vi "F8588A Read Stream.vi"(7 "read timeout [ms] (30000s)":u32=30000, 8 "error in (no error)":errorcluster, 9 "sample size [B]":i32=2, 10 "samples count":i32, 11 "VISA session":refnum<visa-resource-name>) -> (0 "error out":errorcluster, 1 "waveform data int32":i32[](array[numeric]), 2 "waveform data [V]":dbl[](array[numeric]), 3 "dup VISA session":refnum<visa-resource-name>, 4 "scale factor":dbl, 6 "read samples":i32)   [LabVIEW 2020]
doc: "Reads digitized data from memory. If 'Max Read' is set to -1 it reads all available data. It should work with SINt, DINT, SREAL and DREAL modes. ASCII read mode is not finished. It selects the OFORMAT automaticlaly. Data are returned already scaled if transfered in INT."
uses:
  d273381f-8530-47b4-8073-8e484cff5eca.vi
  <vilib>/Utility/error.llb/Error Cluster From Error Code.vi
  <vilib>/ErrorRing/Error Ring.xnode
panel:
  out "reading loop iteration":i32
  out "expected data length (w/o LF)":u32
  out "data length":i32
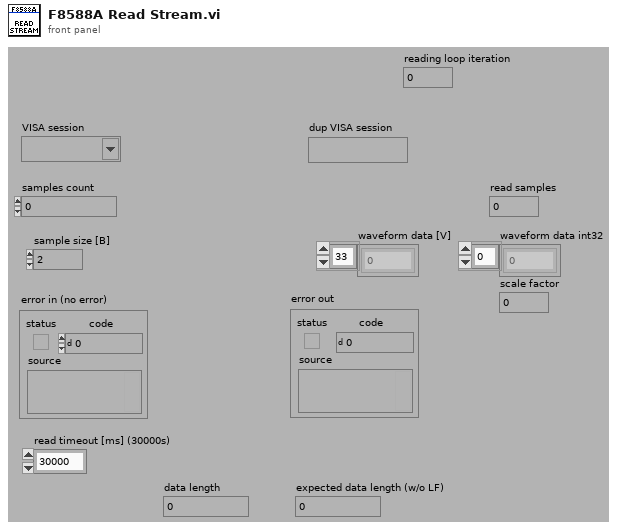
[diagram p1: front panel]
types:
  T1 = enum16{"big-endian, network order", "native, host order", "little-endian"}
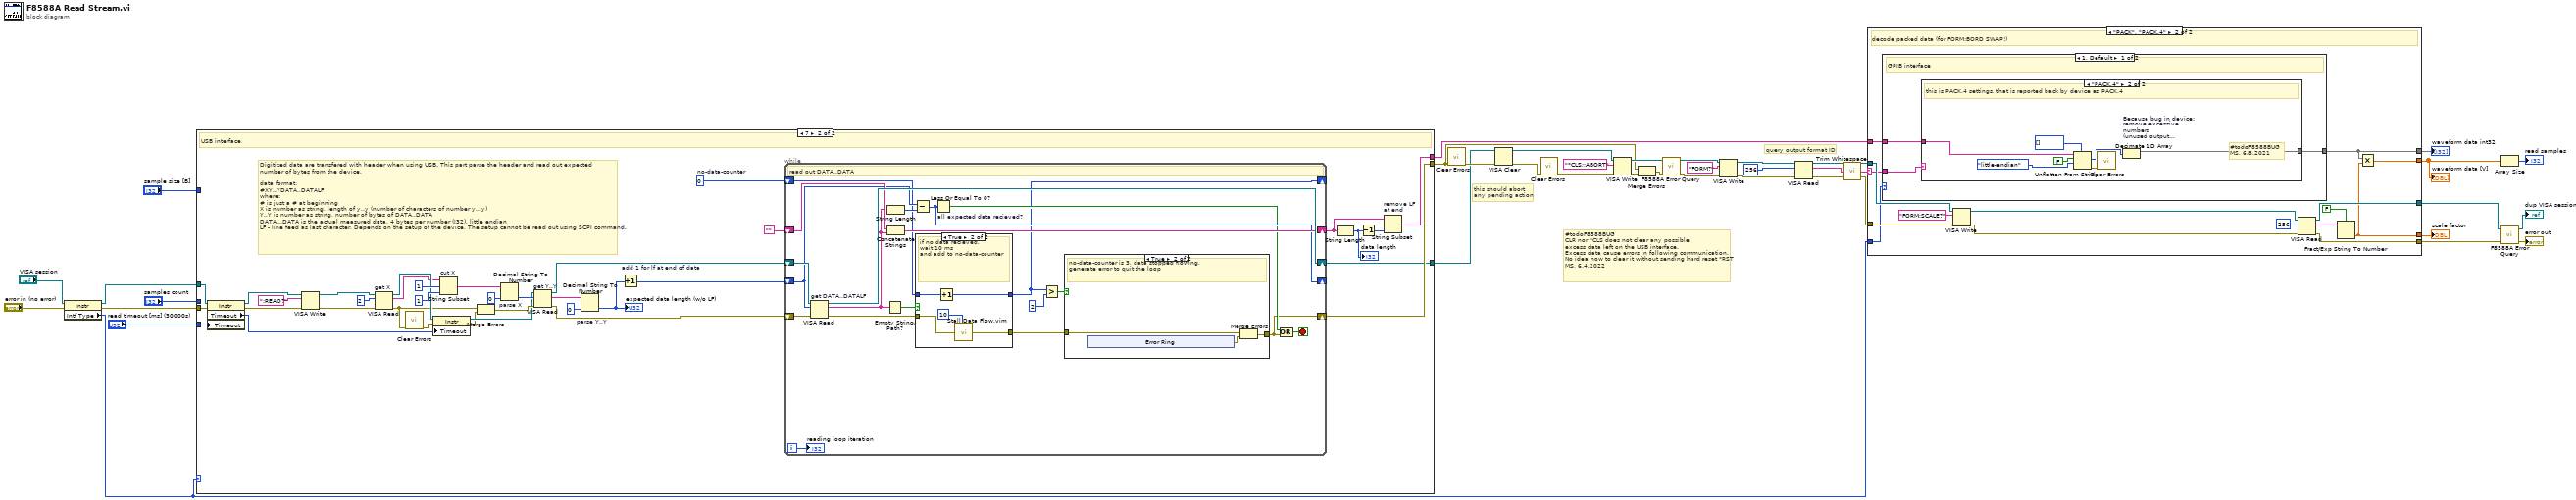
[diagram p0: block diagram]
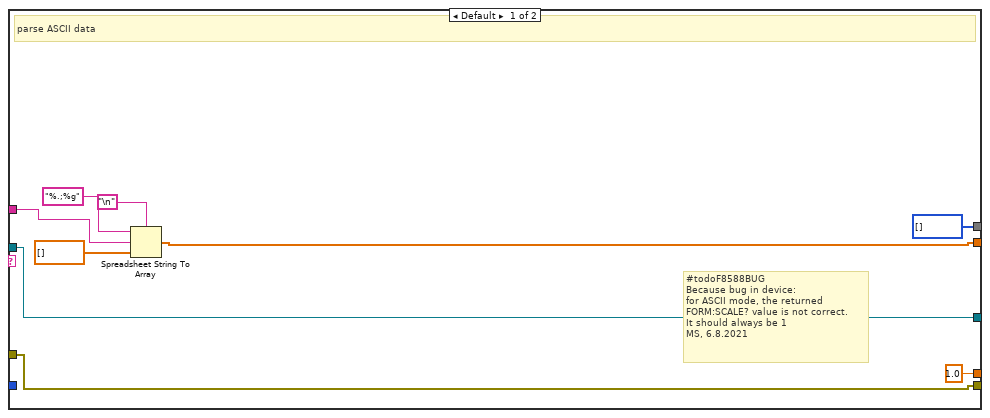
[diagram p2: hidden frame]
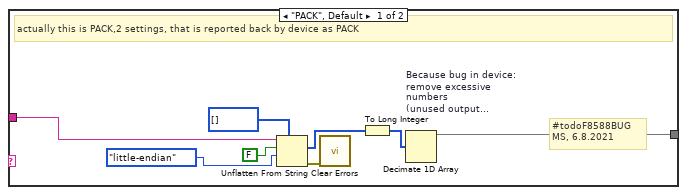
[diagram p3: hidden frame]
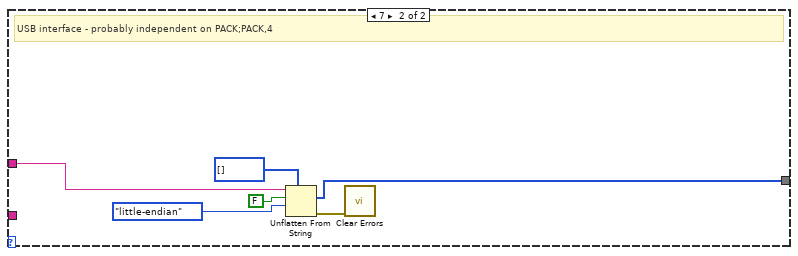
[diagram p4: hidden frame]
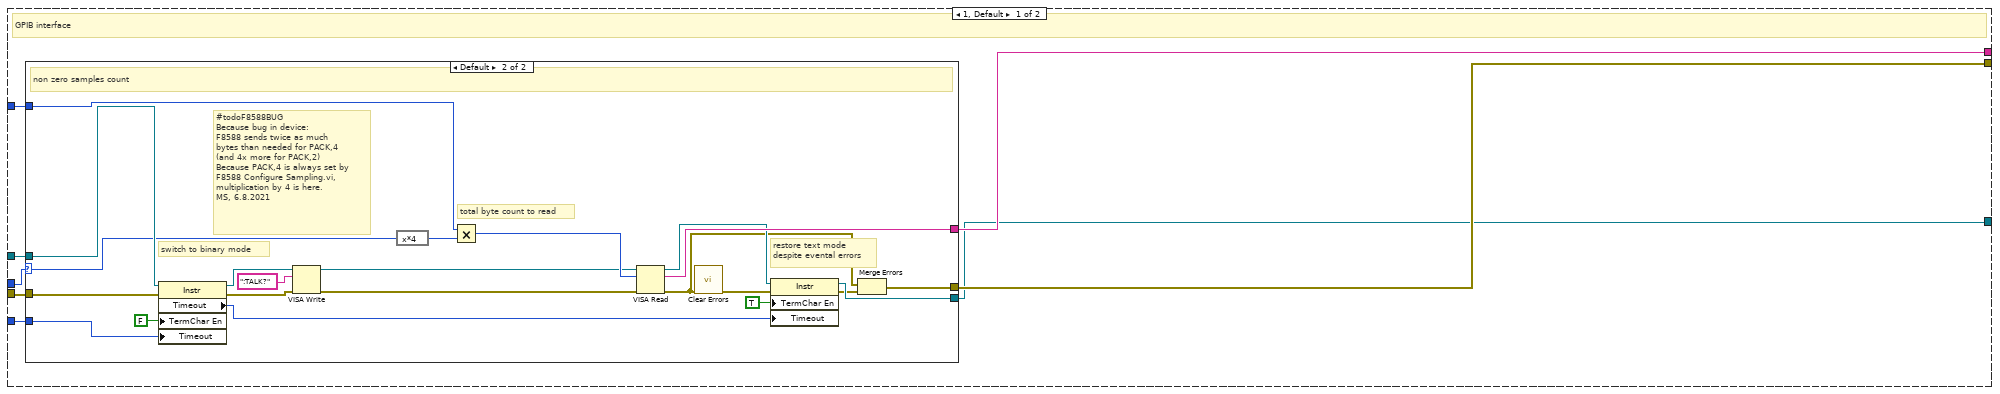
[diagram p5: hidden frame]
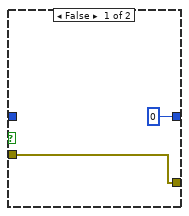
[diagram p8: hidden frame]
diagram:
  # "#todoF8588BUG\nCLR nor *CLS does not clear any possible\nexcess data left on the USB interface.\nExcess data cause errors in following communication.\nNo idea how to clear it without sending hard reset *RST\nMS, 6.4.2022"
  # "query output format ID"
  # "this should abort\nany pending action"
  n1 = property class="Instr"(reference="VISA session", error in="error in (no error)") -> (reference out=w28:refnum<visa-resource-name>, error out=w29:errorcluster, "Intf Type"=w1:u16)
  n2 = case shown="7" w1 {
    tunnel: "read timeout [ms] (30000s)" -> [w45 w87]
    tunnel: w29 -> [w44 w86]
    tunnel: w28 -> [w43 w85]
    tunnel: "samples count" -> [w42 _]
    tunnel: "sample size [B]" -> [w41 _]
    tunnel: [w40 w75] -> w12
    tunnel: [w39 w74] -> w8
    tunnel: [w38 w73] -> w7
    frame 1, Default {
      # "GPIB interface"
      n3 = case shown="Default" w42 {
        selector: w42 -> [_ w49]
        tunnel: w43 -> [w46 w50]
        tunnel: w44 -> [w47 w51]
        tunnel: w41 -> [_ w69]
        tunnel: w45 -> [_ w68]
        tunnel: [w47 w67] -> w39
        tunnel: [w46 w66] -> w38
        tunnel: [_ w65] -> w40
        frame 0 {
        }
        frame Default {
          # "#todoF8588BUG\nBecause bug in device:\nF8588 sends twice as much\nbytes than needed for PACK,4\n(and 4x more for PACK,2)\nBecause PACK,4 is always set by\nF8588 Configure Sampling.vi,\nmultiplication by 4 is here.\nMS, 6.8.2021"
          # "restore text mode\ndespite evental errors"
          # "switch to binary mode"
          # "total byte count to read"
          # "non zero samples count"
          n4 = property on="Property Node" class="Instr"(reference=w50, error in=w51, "TermChar En"=FALSE, "Timeout"=w68) -> (reference out=w54:refnum<visa-resource-name>, error out=w55:errorcluster, "Timeout"=w60:u32)
          n5 = VISA Write(VISA resource name=w54, write buffer=":TALK?", error in (no error)=w55) -> (VISA resource name out=w52:refnum<visa-resource-name>, error out=w53:errorcluster)  [unwired: 1 out]
          n6 = expression code="x*4"(w49) -> (w48:i32)
          n7 = Multiply(x=w69, y=w48) -> (x*y=w64:i32)
          n8 = VISA Read(VISA resource name=w52, byte count=w64, error in (no error)=w53) -> (VISA resource name out=w61:refnum<visa-resource-name>, read buffer=w65:string, error out=w57:errorcluster)  [unwired: 1 out]
          n9 = call <vilib>:"Clear Errors.vi"("error in (no error)"=w57) -> ("error out"=w59:errorcluster)  [unwired: 5 in, 1 out]
          n10 = property class="Instr"(reference=w61, error in=w59, "TermChar En"=TRUE, "Timeout"=w60) -> (reference out=w66:refnum<visa-resource-name>, error out=w58:errorcluster)
          n11 = Merge Errors(w57, w58) -> (w67:errorcluster)
        }
      }
    }
    frame 7 {
      w70 = u32 0  # no-data-counter
      # "Digitized data are transfered with header when using USB. This part parse the header and read out expected\nnumber of bytes from the device.\n\ndata format:\n#XY..YDATA..DATALF\nwhere:\n# is just a # at beginning\nX is number as string, length of y..y (number of characters of number y...y)\nY..Y is number as string, number of bytes of DATA..DATA\nDATA...DATA is the actual measured data, 4 bytes per number (I32), little endian\nLF - line feed as last character. Depends on the setup of the device. The setup cannot be read out using SCPI command."
      # "USB interface"
      n12 = property on="Property Node" class="Instr"(reference=w85, error in=w86, "Timeout"=w87) -> (reference out=w91:refnum<visa-resource-name>, error out=w92:errorcluster, "Timeout"=w94:u32)
      n13 = VISA Write(VISA resource name=w91, write buffer=":READ?", error in (no error)=w92) -> (VISA resource name out=w89:refnum<visa-resource-name>, error out=w90:errorcluster)  [unwired: 1 out]
      n14 = VISA Read "get X"(VISA resource name=w89, byte count=u32 2, error in (no error)=w90) -> (VISA resource name out=w95:refnum<visa-resource-name>, read buffer=w81:string, error out=w93:errorcluster)  [unwired: 1 out]
      n15 = call <vilib>:"Clear Errors.vi"("error in (no error)"=w93) -> ("error out"=w72:errorcluster)  [unwired: 5 in, 1 out]
      n16 = property class="Instr"(reference=w95, error in=w72, "Timeout"=w94) -> (reference out=w82:refnum<visa-resource-name>, error out=w71:errorcluster)
      n17 = String Subset "cut X"(string=w81, offset (0)=1, length (rest)=1 ("length (rest)")) -> (substring=w103:string)
      n18 = Merge Errors(w93, w71) -> (w83:errorcluster)
      n19 = Decimal String To Number "parse X"(string=w103, default (0L)=u32 0 ("default (0 I32)")) -> (number=w101:u32)  [unwired: 1 in, 1 out]
      n20 = VISA Read "get Y..Y"(VISA resource name=w82, byte count=w101, error in (no error)=w83) -> (VISA resource name out=w97:refnum<visa-resource-name>, read buffer=w80:string, error out=w96:errorcluster)  [unwired: 1 out]
      n21 = Decimal String To Number "parse Y..Y"(string=w80, default (0L)=u32 0 ("default (0 I32)")) -> (number=w99:u32)  [unwired: 1 in, 1 out]
      "expected data length (w/o LF)" <- w99
      n22 = Increment "add 1 for lf at end of data"(x=w99) -> (x+1=w98:u32)
      n23 = while {
        shift-right: [w123] -> w73
        shift-left: w97 -> [w125]
        shift-right: [w107] -> w74
        shift-left: w96 -> [w124]
        shift-right: [w119] -> _
        shift-left: w98 -> [w120]
        shift-right: [w121] -> w77
        shift-left: "" -> [w122]
        shift-right: [w111] -> _
        shift-left: w70 -> [w112]
        i -> [w106]
        stop <- w117 stop-if-true
        # "read out DATA..DATA"
        n24 = VISA Read "get DATA..DATALF"(VISA resource name=w125, byte count=w120, error in (no error)=w124) -> (VISA resource name out=w123:refnum<visa-resource-name>, read buffer=w115:string, error out=w114:errorcluster)  [unwired: 1 out]
        n25 = Empty String/Path?(string/path=w115) -> (empty?=w113:bool)
        n26 = String Length(string=w115) -> (length=w118:i32)
        n27 = Concatenate Strings(w122, w115) -> (w121:string)
        n28 = Subtract(x=w120, y=w118) -> (x-y=w119:u32)
        n29 = case shown="True" w113 {
          tunnel: w114 -> [w136 w141]
          tunnel: [w136 w140] -> w108
          tunnel: w112 -> [_ w138]
          tunnel: [u32 0 ("x+1") w137] -> w111
          frame False {
          }
          frame True {
            # "if no data recieved,\nwait 10 ms\nand add to no-data-counter"
            n30 = Increment(x=w138) -> (x+1=w137:u32)
            n31 = call "Stall Data Flow.vim"("value in"=w141, "milliseconds to wait"=u32 10) -> ("value out"=w140:errorcluster)  [unwired: 1 out]
          }
        }
        n32 = Less Or Equal To 0? "all expected data recieved?"(x=w119) -> (x <= 0?=w116:bool)
        n33 = Greater?(x=w111, y=u32 2 ("x")) -> (0:w109:bool)
        n34 = case shown="True" w109 {
          tunnel: w108 -> [w126 w128]
          tunnel: [w126 w127] -> w107
          frame False {
          }
          frame True {
            # "no-data-counter is 3, data stopped flowing,\ngenerate error to quit the loop"
            n35 = xnode "Error Ring"() -> ("error out"=w129:errorcluster)
            n36 = Merge Errors(w128, w129) -> (w127:errorcluster)
          }
        }
        n37 = Compound Arithmetic op=OR(w116, w107) -> (w117:bool)
        "reading loop iteration" <- w106
      }
      n38 = String Length(string=w77) -> (length=w76:i32)
      "data length" <- w76
      n39 = Decrement(x=w76) -> (x-1=w79:i32)
      n40 = String Subset "remove LF\nat end"(string=w77, length (rest)=w79) -> (substring=w75:string)  [unwired: 1 in]
    }
  }
  n41 = call <vilib>:"Clear Errors.vi"("error in (no error)"=w8) -> ("error out"=w13:errorcluster)  [unwired: 5 in, 1 out]
  n42 = VISA Clear(VISA resource name=w7, error in (no error)=w13) -> (VISA resource name out=w16:refnum<visa-resource-name>, error out=w14:errorcluster)
  n43 = call <vilib>:"Clear Errors.vi"("error in (no error)"=w14) -> ("error out"=w15:errorcluster)  [unwired: 5 in, 1 out]
  n44 = VISA Write(VISA resource name=w16, write buffer="*CLS;:ABORT", error in (no error)=w15) -> (VISA resource name out=w21:refnum<visa-resource-name>, error out=w17:errorcluster)  [unwired: 1 out]
  n45 = Merge Errors(w8, w17) -> (w20:errorcluster)
  n46 = call "F8588A Error Query.vi"("error in (no error)"=w20, "VISA resource name"=w21) -> ("error out"=w22:errorcluster, "VISA resource name out"=w23:refnum<visa-resource-name>)  [unwired: 6 in, 2 out]
  n47 = VISA Write(VISA resource name=w23, write buffer="FORM?", error in (no error)=w22) -> (VISA resource name out=w19:refnum<visa-resource-name>, error out=w18:errorcluster)  [unwired: 1 out]
  n48 = VISA Read(VISA resource name=w19, byte count=u32 256, error in (no error)=w18) -> (VISA resource name out=w27:refnum<visa-resource-name>, read buffer=w24:string, error out=w26:errorcluster)  [unwired: 1 out]
  n49 = call <vilib>:"Trim Whitespace.vi"("string"=w24) -> ("trimmed string"=w25:string)  [unwired: 1 in]
  n50 = case shown="\"PACK\", \"PACK,4\"" w25 {
    selector: w25 -> [_ w155]
    tunnel: [w149 w162] -> w6
    tunnel: [w150 w161] -> w5
    tunnel: w27 -> [w150 w160]
    tunnel: w26 -> [w149 w159]
    tunnel: [1.0 w157] -> w4
    tunnel: w12 -> [w144 w156]
    tunnel: [w143 w154] -> w3
    tunnel: [i32[] [] w152] -> w2
    tunnel: w1 -> [_ w151]
    frame Default {
      # "#todoF8588BUG\nBecause bug in device:\nfor ASCII mode, the returned\nFORM:SCALE? value is not correct.\nIt should always be 1\nMS, 6.8.2021"
      # "parse ASCII data"
      n51 = Spreadsheet String To Array(delimiter (Tab)="\n", format string="%.;%g", spreadsheet string=w144, array type (2D Dbl)=dbl[] []) -> (array=w143:dbl[])
    }
    frame "PACK", "PACK,4" {
      # "decode packed data (for FORM:BORD SWAP!)"
      n52 = case shown="1, Default" w151 {
        tunnel: w156 -> [w169 w187]
        tunnel: w155 -> [w168 _]
        tunnel: [w167 w186] -> w152
        frame 1, Default {
          # "GPIB interface"
          n53 = case shown="\"PACK,4\"" w168 {
            tunnel: w169 -> [w177 w184]
            tunnel: [w171 w179] -> w167
            frame "PACK", Default {
              # "#todoF8588BUG\nMS, 6.8.2021"
              # "actually this is PACK,2 settings, that is reported back by device as PACK"
              n54 = Unflatten From String(type=i16[] [], binary string=w177, data includes array or string size? (T)=FALSE, byte order (0:big-endian, network order)=T1."little-endian") -> (value=w173:i16[], error out=w170:errorcluster)  [unwired: 1 in, 1 out]
              n55 = call <vilib>:"Clear Errors.vi"("error in (no error)"=w170) -> ()  [unwired: 5 in, 2 out]
              n56 = To Long Integer(number=w173) -> (32bit integer=w172:i32[])
              n57 = Decimate 1D Array "Because bug in device:\nremove excessive\nnumbers\n(unused output\nterminals are important!)"(w172) -> (w171:i32[])  [unwired: 3 out]
            }
            frame "PACK,4" {
              # "#todoF8588BUG\nMS, 6.8.2021"
              # "this is PACK,4 settings, that is reported back by device as PACK,4"
              n58 = Unflatten From String(type=i32[] [], binary string=w184, data includes array or string size? (T)=FALSE, byte order (0:big-endian, network order)=T1."little-endian") -> (value=w180:i32[], error out=w178:errorcluster)  [unwired: 1 in, 1 out]
              n59 = call <vilib>:"Clear Errors.vi"("error in (no error)"=w178) -> ()  [unwired: 5 in, 2 out]
              n60 = Decimate 1D Array "Because bug in device:\nremove excessive\nnumbers\n(unused output\nterminals are important!)"(w180) -> (w179:i32[])  [unwired: 1 out]
            }
          }
        }
        frame 7 {
          # "USB interface - probably independent on PACK;PACK,4"
          n61 = Unflatten From String(type=i32[] [], binary string=w187, data includes array or string size? (T)=FALSE, byte order (0:big-endian, network order)=T1."little-endian") -> (value=w186:i32[], error out=w185:errorcluster)  [unwired: 1 in, 1 out]
          n62 = call <vilib>:"Clear Errors.vi"("error in (no error)"=w185) -> ()  [unwired: 5 in, 2 out]
        }
      }
      n63 = VISA Write(VISA resource name=w160, write buffer="FORM:SCALE?", error in (no error)=w159) -> (VISA resource name out=w164:refnum<visa-resource-name>, error out=w153:errorcluster)  [unwired: 1 out]
      n64 = VISA Read(VISA resource name=w164, byte count=u32 256, error in (no error)=w153) -> (VISA resource name out=w161:refnum<visa-resource-name>, read buffer=w158:string, error out=w162:errorcluster)  [unwired: 1 out]
      n65 = Fract/Exp String To Number(use system decimal point (T)=FALSE, string=w158) -> (number=w157:dbl)  [unwired: 2 in, 1 out]
      n66 = Multiply(x=w152, y=w157) -> (x*y=w154:dbl[])
    }
  }
  "waveform data [V]" <- w3
  "waveform data int32" <- w2
  "scale factor" <- w4
  n67 = Array Size(array=w3) -> (size(s)=→"read samples":i32)
  n68 = call "F8588A Error Query.vi"("error in (no error)"=w6, "VISA resource name"=w5) -> ("error out"=→"error out":errorcluster, "VISA resource name out"=→"dup VISA session":refnum<visa-resource-name>)  [unwired: 6 in, 2 out]
